vi "Convert Old CAN Log to XNET.vi"() -> ()   [LabVIEW 2014]
uses:
  <vilib>/RioEmbeddedCAN/RioEmbeddedCAN.llb/CANFrameControl.ctl
panel:
  in  "New File path":path
  in  "Source":path=path "C:/Data for Processing/150215 132046.tdms"
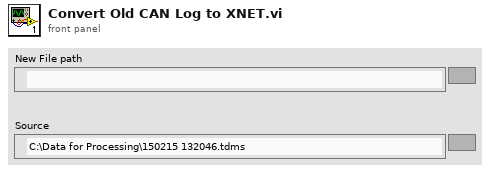
[diagram p1: front panel]
types:
  T1 = enum16{"big-endian, network order", "native, host order", "little-endian"}
  T2 = enum16{"open", "open or create", "create or replace", "create", "open (read-only)"}
  T3 = typedef "CANFrameControl.ctl" = cluster{"identifier":u32, "extended?":bool, "type":u8, "payload":u8[]}
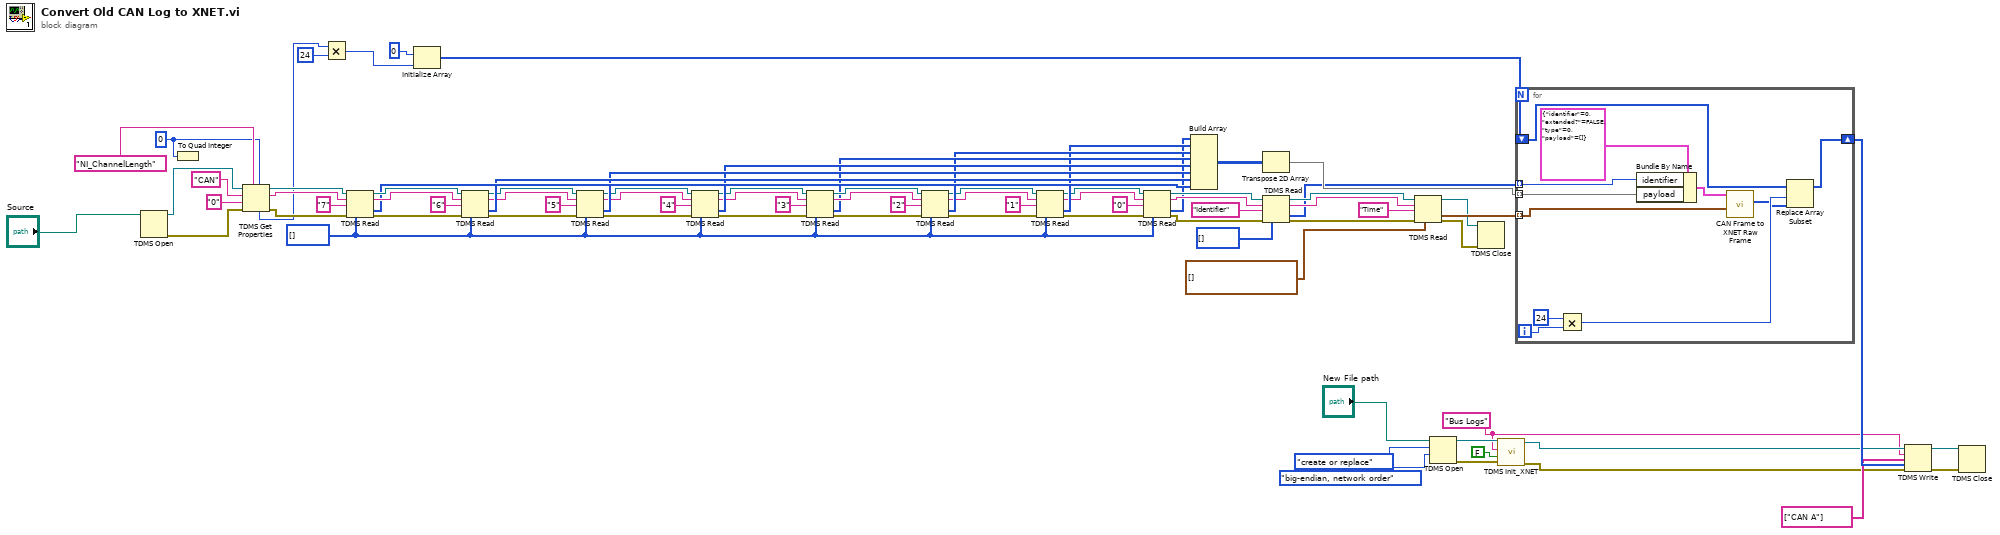
[diagram p0: block diagram]
diagram:
  w2 = "Bus Logs" ("group name")
  w26 = u8[] []
  w76 = u64 0 ("data type")
  n1 = TDMS Open(11:"Source") -> (0:w81:errorcluster, 3:w82:refnum<k34>)  [unwired: 6 in]
  n2 = To Quad Integer(1:w76) -> ()  [unwired: 1 out]
  n3 = TDMS Get Properties(5:w76, 7:"NI_ChannelLength" ("property name"), 8:w81, 9:"0" ("channel name"), 10:"CAN" ("group name"), 11:w82) -> (0:w74:errorcluster, 2:w73:string, 3:w75:refnum<k34>, 4:w18:u64)  [unwired: 2 out]
  n4 = Multiply(x=w18, y=u64 24) -> (x*y=w16:u64)
  n5 = TDMS Read(0:w75, 5:w73, 7:"7" ("channel name(s) in"), 11:w74, 12:w26) -> (4:w71:refnum<k34>, 6:w69:string, 10:w67:u8[], 15:w70:errorcluster)  [unwired: 3 in, 2 out]
  n6 = Initialize Array(u8 0, w16) -> (w14:u8[])
  n7 = TDMS Read(0:w71, 5:w69, 7:"6" ("channel name(s) in"), 11:w70, 12:w26) -> (4:w65:refnum<k34>, 6:w63:string, 10:w66:u8[], 15:w64:errorcluster)  [unwired: 3 in, 2 out]
  n8 = TDMS Read(0:w65, 5:w63, 7:"5" ("channel name(s) in"), 11:w64, 12:w26) -> (4:w60:refnum<k34>, 6:w59:string, 10:w61:u8[], 15:w57:errorcluster)  [unwired: 3 in, 2 out]
  n9 = TDMS Read(0:w60, 5:w59, 7:"4" ("channel name(s) in"), 11:w57, 12:w26) -> (4:w55:refnum<k34>, 6:w53:string, 10:w56:u8[], 15:w54:errorcluster)  [unwired: 3 in, 2 out]
  n10 = TDMS Read(0:w55, 5:w53, 7:"3" ("channel name(s) in"), 11:w54, 12:w26) -> (4:w51:refnum<k34>, 6:w49:string, 10:w46:u8[], 15:w50:errorcluster)  [unwired: 3 in, 2 out]
  n11 = TDMS Read(0:w51, 5:w49, 7:"2" ("channel name(s) in"), 11:w50, 12:w26) -> (4:w28:refnum<k34>, 6:w22:string, 10:w45:u8[], 15:w27:errorcluster)  [unwired: 3 in, 2 out]
  n12 = TDMS Read(0:w28, 5:w22, 7:"1" ("channel name(s) in"), 11:w27, 12:w26) -> (4:w21:refnum<k34>, 6:w19:string, 10:w25:u8[], 15:w20:errorcluster)  [unwired: 3 in, 2 out]
  n13 = TDMS Read(0:w21, 5:w19, 7:"0" ("channel name(s) in"), 11:w20, 12:w26) -> (4:w44:refnum<k34>, 6:w42:string, 10:w24:u8[], 15:w43:errorcluster)  [unwired: 3 in, 2 out]
  n14 = Build Array(w24, w25, w45, w46, w56, w61, w66, w67) -> (w34:u8[][])
  n15 = Transpose 2D Array(2D array=w34) -> (transposed array=w33:u8[][])
  n16 = TDMS Read(0:w44, 5:w42, 7:"Identifier" ("channel name(s) in"), 11:w43, 12:u32[] []) -> (4:w39:refnum<k34>, 6:w37:string, 10:w31:u32[], 15:w38:errorcluster)  [unwired: 3 in, 2 out]
  n17 = TDMS Read(0:w39, 5:w37, 7:"Time" ("channel name(s) in"), 11:w38, 12:timestamp[] []) -> (4:w30:refnum<k34>, 10:w32:timestamp[], 15:w29:errorcluster)  [unwired: 3 in, 3 out]
  n18 = TDMS Open(9:T1."big-endian, network order" ("byte order (2:little-endian)"), 10:T2."create or replace" ("operation (0:open)"), 11:"New File path") -> (0:w5:errorcluster, 3:w6:refnum<k34>)  [unwired: 4 in]
  n19 = TDMS Close(8:w29, 11:w30) -> ()  [unwired: 2 out]
  n20 = call "TDMS Init_XNET.vi"("error in (no error)"=w5, "sbRIO?"=FALSE, "group name"=w2, "tdms file"=w6) -> ("error out"=w3:errorcluster, "tdms file out"=w4:refnum<k34>)  [unwired: 6 in]
  n21 = for {
    tunnel: w33 -> [w92] mode=indexing
    tunnel: w32 -> [w89] mode=indexing
    tunnel: w31 -> [w91] mode=indexing
    shift-right: [w87] -> w12
    shift-left: w14 -> [w88]
    i -> [w86]
    n22 = Multiply(x=24, y=w86) -> (x*y=w84:i32)
    n23 = Bundle By Name(cluster=T3 {"identifier"=0, "extended?"=FALSE, "type"=0, "payload"=[]} ("CAN frame"), "identifier"=w91, "payload"=w92) -> (w90:T3)
    n24 = call "CAN Frame to XNET Raw Frame.vi"("timestamp"=w89, "CAN frame"=w90) -> ("Raw Frame"=w83:u8[])  [unwired: 8 in, 1 out]
    n25 = Replace Array Subset(array=w88, new element=w83, index=w84) -> (w87:u8[])
  }
  n26 = TDMS Write(0:w4, 5:w2, 7:string[] ["CAN A"] ("channel name(s) in (Untitled)"), 9:w12, 11:w3) -> (4:w10:refnum<k34>, 15:w9:errorcluster)  [unwired: 1 in, 2 out]
  n27 = TDMS Close(8:w9, 11:w10) -> ()  [unwired: 2 out]
